vi "Intake.vi"(2 "Rollers Control":bool, 3 "Pneumatics Extended":bool, 4 "Tote Sensor":bool) -> (0 "Pneumatics":bool, 1 "Rollers":bool)   [LabVIEW 2014]
panel:
  out "State":T1(ring)
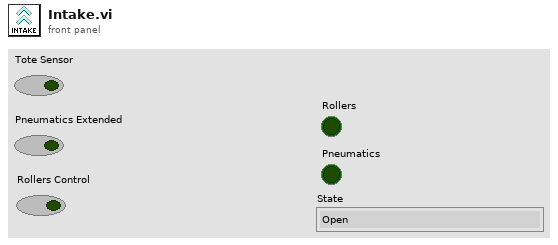
[diagram p1: front panel]
types:
  T1 = enum16{"Open", "Shut Rolling", "Shut Not Rolling"}
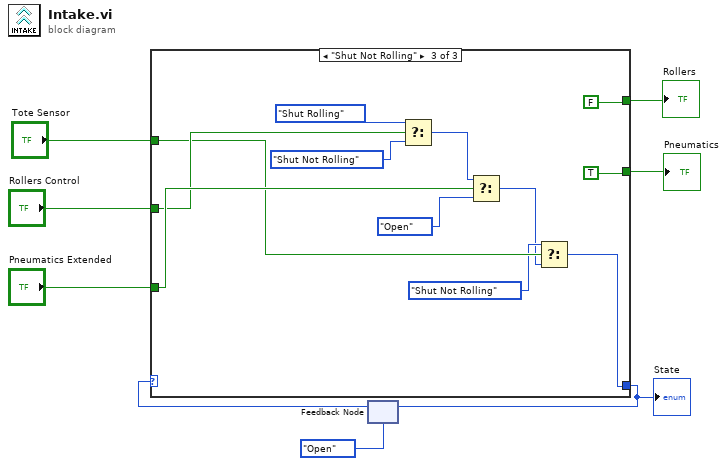
[diagram p0: block diagram]
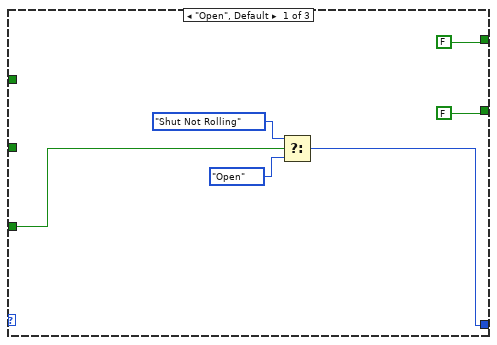
[diagram p2: hidden frame]
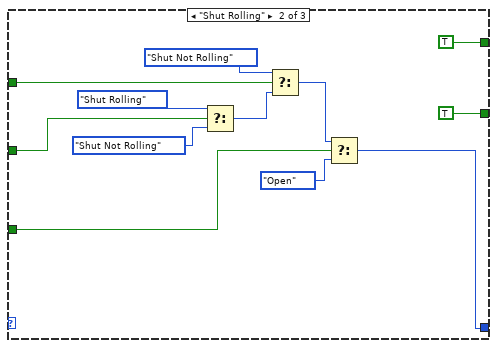
[diagram p3: hidden frame]
diagram:
  n1 = feedback #1(T1."Open" ("State")) -> (w8:T1)
  n2 = case shown="\"Shut Not Rolling\"" w8 {
    tunnel: [w14 w22 w29] -> w7
    tunnel: "Tote Sensor" -> [_ w21 w30]
    tunnel: "Rollers Control" -> [_ w25 w35]
    tunnel: "Pneumatics Extended" -> [w13 w26 w36]
    tunnel: [FALSE TRUE FALSE] -> w3
    tunnel: [FALSE TRUE TRUE] -> w2
    frame "Open", Default {
      n3 = Select(t=T1."Shut Not Rolling" ("State"), s=w13, f=T1."Open" ("t")) -> (s? t:f=w14:T1)
    }
    frame "Shut Rolling" {
      n4 = Select(t=T1."Shut Rolling", s=w25, f=T1."Shut Not Rolling" ("State")) -> (s? t:f=w20:T1)
      n5 = Select(t=T1."Shut Not Rolling", s=w21, f=w20) -> (s? t:f=w15:T1)
      n6 = Select(t=w15, s=w26, f=T1."Open" ("t")) -> (s? t:f=w22:T1)
    }
    frame "Shut Not Rolling" {
      n7 = Select(t=T1."Shut Rolling", s=w35, f=T1."Shut Not Rolling" ("State")) -> (s? t:f=w31:T1)
      n8 = Select(t=w31, s=w36, f=T1."Open" ("t")) -> (s? t:f=w27:T1)
      n9 = Select(t=T1."Shut Not Rolling" ("f"), s=w30, f=w27) -> (s? t:f=w29:T1)
    }
  }
  "Rollers" <- w3
  "Pneumatics" <- w2
  "State" <- w7
  n10 = feedback-in #1(w7) -> ()
